vi "CheckLic.vi"() -> (0 "数据保存":bool, 1 "强制操作":bool, 2 "LicCode":string, 3 "机器码":string, 4 "参数生成":bool, 5 "参数配置":bool, 8 "鉴权通过":bool)   [LabVIEW 2013]
panel:
  out "子字符串":string
  out "Tip":string
  out "注册码":string
  out "连接的字符串":string
  in  "退出":bool
  in  "注册":bool
  in  "簇":T1
  out "字符串":string
  out "Times":dbl
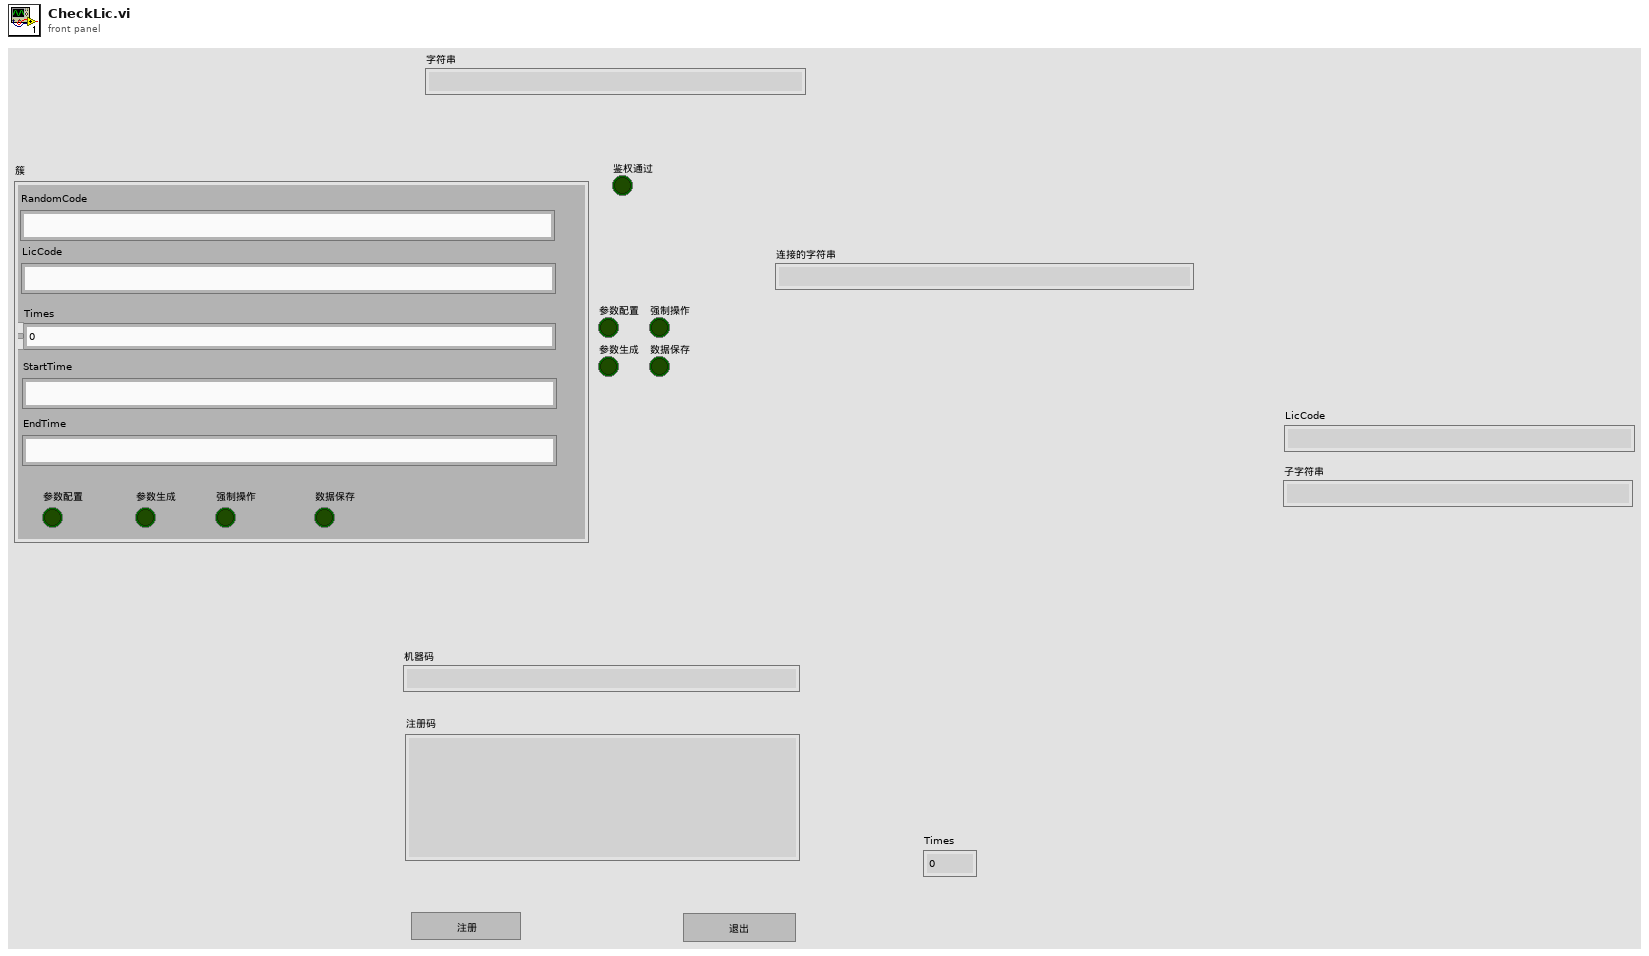
[diagram p1: front panel]
types:
  T1 = cluster{"RandomCode":string, "LicCode":string, "Times":dbl, "StartTime":string, "EndTime":string, "参数配置":bool, "参数生成":bool, "强制操作":bool, "数据保存":bool}
  T2 = enum32{"Invalid", "Standard", "Closed", "Hidden", "Minimized", "Maximized"}
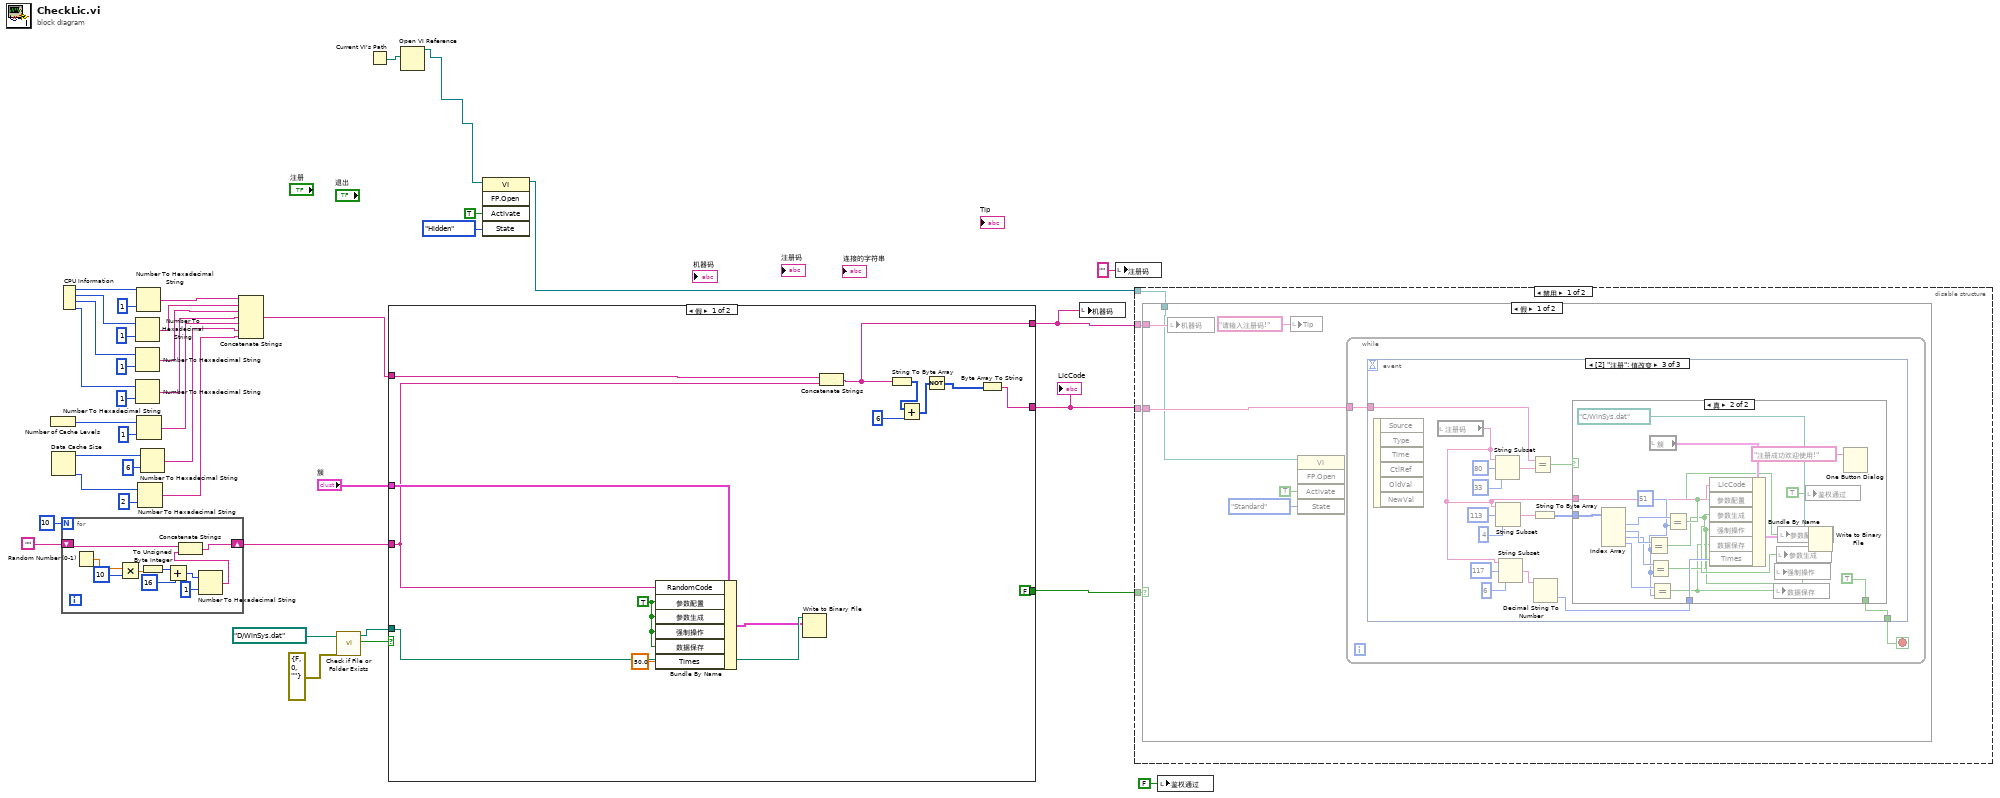
[diagram p0: block diagram]
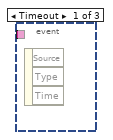
[diagram p2: hidden frame]
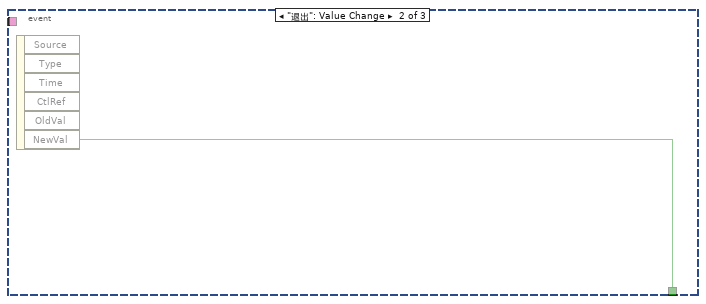
[diagram p3: hidden frame]
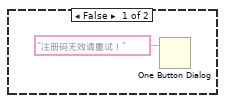
[diagram p4: hidden frame]
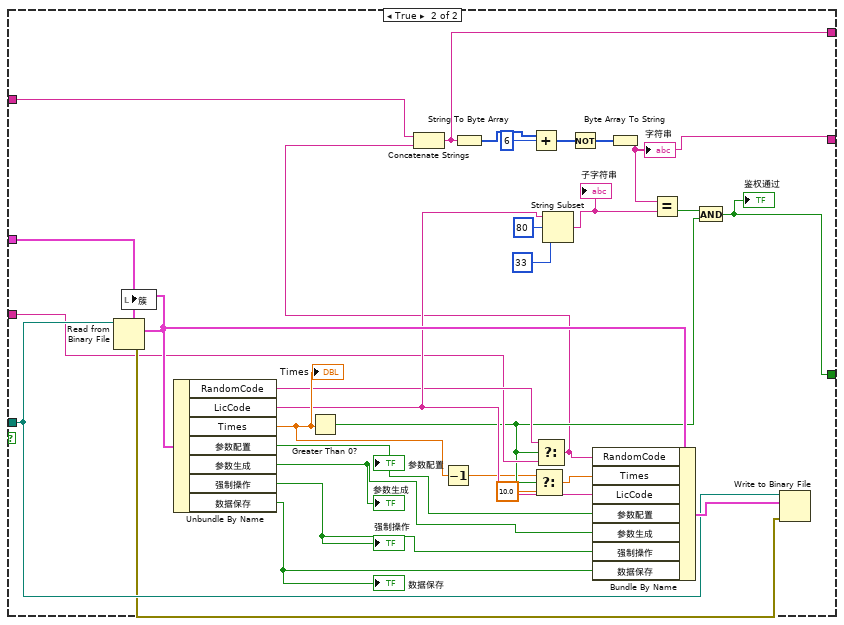
[diagram p7: hidden frame]
diagram:
  n1 = Number of Cache Levels() -> (w25:i32)
  n2 = Data Cache Size() -> (4:w26:i32, 7:w28:i32)  [unwired: 1 in]
  n3 = CPU Information() -> (4:w16:i32, 5:w20:i32, 6:w21:i32, 7:w22:i32)
  n4 = for {
    N: 10 -> [_]
    shift-right: [w42] -> w1
    shift-left: "" -> [w43]
    n5 = Random Number (0-1)() -> (number: 0 to 1=w50:dbl)
    n6 = Multiply(x=w50, y=u8 10) -> (x*y=w48:dbl)
    n7 = To Unsigned Byte Integer(number=w48) -> (unsigned 8bit integer=w46:u8)
    n8 = Add(x=w46, y=u8 16) -> (x+y=w44:u8)
    n9 = Number To Hexadecimal String(1:i16 1 ("宽度(-)"), 2:w44) -> (0:w41:string)
    n10 = Concatenate Strings(w43, w41) -> (w42:string)
  }
  n11 = Number To Hexadecimal String(1:i16 1 ("宽度(-)"), 2:w20) -> (0:w30:string)
  n12 = Number To Hexadecimal String(1:i16 1 ("宽度(-)"), 2:w21) -> (0:w31:string)
  n13 = Number To Hexadecimal String(1:i16 1 ("宽度(-)"), 2:w22) -> (0:w32:string)
  n14 = Number To Hexadecimal String(1:i16 1 ("宽度(-)"), 2:w16) -> (0:w29:string)
  n15 = Number To Hexadecimal String(1:i16 1 ("宽度(-)"), 2:w25) -> (0:w33:string)
  n16 = Number To Hexadecimal String(1:i16 2 ("宽度(-)"), 2:w28) -> (0:w35:string)
  n17 = Number To Hexadecimal String(1:i16 6 ("宽度(-)"), 2:w26) -> (0:w34:string)
  n18 = Concatenate Strings(w29, w30, w31, w32, w33, w34, w35) -> (w14:string)
  n19 = call <vilib>:"Check if File or Folder Exists.vi"("error in (no error)"=errorcluster {"status"=FALSE, "code"=0, "source"=""}, "path"=path "D:/WinSys.dat" ("文件（使用对话框）")) -> ("file or folder exists?"=w38:bool, "dup path"=w37:path)  [unwired: 7 in, 1 out]
  n20 = Current VI's Path() -> (path=w10:path)
  n21 = case shown="假" w38 {
    tunnel: w37 -> [w63 w79]
    tunnel: "簇" -> [w61 w92]
    tunnel: w14 -> [w58 w89]
    tunnel: [FALSE w83] -> w13
    tunnel: [w54 w82] -> w12
    tunnel: [w53 w81] -> w5
    tunnel: w1 -> [w52 w69]
    frame False {
      w60 = TRUE ("参数配置")
      n22 = Bundle By Name(cluster=w61, "RandomCode"=w52, "参数配置"=w60, "参数生成"=w60, "强制操作"=w60, "数据保存"=w60, "Times"=50.0) -> (w62:T1)
      n23 = Write to Binary File(file (use dialog)=w63, data=w62) -> ()  [unwired: 4 in, 3 out]
      n24 = Concatenate Strings(w58, w52) -> (w53:string)
      n25 = String To Byte Array(string=w53) -> (unsigned byte array=w57:u8[])
      n26 = Add(x=w57, y=u8 6) -> (x+y=w55:u8[])
      n27 = Not(x=w55) -> ()  [unwired: 1 out]
      n28 = Byte Array To String(unsigned byte array=w55) -> (string=w54:string)
    }
    frame True {
      n29 = Read from Binary File(5:w92, 11:w79) -> (0:w71:errorcluster, 2:w78:T1)  [unwired: 4 in, 2 out]
      n30 = local write "簇"(w78) -> ()
      n31 = Unbundle By Name(w78) -> ("RandomCode"=w70:string, "LicCode"=w72:string, "Times"=w77:dbl, "参数配置"=w76:bool, "参数生成"=w75:bool, "强制操作"=w74:bool, "数据保存"=w73:bool)
      "参数配置" <- w76
      "参数生成" <- w75
      "强制操作" <- w74
      "数据保存" <- w73
      "Times" <- w77
      n32 = Greater Than 0?(x=w77) -> (x > 0?=w68:bool)
      n33 = Decrement(x=w77) -> (x-1=w66:dbl)
      n34 = Select(t=w66, s=w68, f=10.0) -> (s? t:f=w67:dbl)
      n35 = Select(t=w70, s=w68, f=w69) -> (s? t:f=w64:string)
      n36 = Concatenate Strings(w89, w64) -> (w81:string)
      n37 = String To Byte Array(string=w81) -> (unsigned byte array=w88:u8[])
      n38 = Add(x=w88, y=u8 6) -> (x+y=w86:u8[])
      n39 = String Subset(string=w72, offset (0)=80 ("偏移量(0)"), length (rest)=33 ("长度（剩余）")) -> (substring=w85:string)
      "子字符串" <- w85
      n40 = Not(x=w86) -> ()  [unwired: 1 out]
      n41 = Bundle By Name(cluster=w78, "RandomCode"=w64, "Times"=w67, "LicCode"=w72, "参数配置"=w76, "参数生成"=w75, "强制操作"=w74, "数据保存"=w73) -> (w80:T1)
      n42 = Byte Array To String(unsigned byte array=w86) -> (string=w82:string)
      "字符串" <- w82
      n43 = Equal?(x=w82, y=w85) -> (x = y?=w84:bool)
      n44 = And(x=w84, y=w68) -> (x .and. y?=w83:bool)
      "鉴权通过" <- w83
      n45 = Write to Binary File(file (use dialog)=w79, data=w80, error in=w71) -> ()  [unwired: 3 in, 3 out]
    }
  }
  "LicCode" <- w12
  n46 = Open VI Reference(vi path=w10) -> (vi reference=w7:refnum<vi>)  [unwired: 5 in, 1 out]
  n47 = invoke class="VI" method="FP.Open"(reference=w7, "Activate"=TRUE ("激活？"), "State"=T2."Hidden" ("状态")) -> (reference out=w6:refnum<vi>)  [unwired: 2 in, 4 out]
  n48 = local write "机器码"(w5) -> ()
  n49 = local write "注册码"("" ("注册码")) -> ()
  n50 = disable-structure shown="禁用" {
    disable-tunnel: w13 -> [w96 _]
    disable-tunnel: w12 -> [w95 _]
    disable-tunnel: w5 -> [w94 _]
    disable-tunnel: w6 -> [w93 _]
    frame Disabled {
      n51 = case shown="假" w96 {
        tunnel: w95 -> [w102 _]
        tunnel: w94 -> [w100 _]
        tunnel: w93 -> [w97 _]
        frame False {
          n52 = local write "机器码"(w100) -> ()
          n53 = local write "Tip"("请输入注册码!" ("Tip")) -> ()
          n54 = invoke class="VI" method="FP.Open"(reference=w97, "Activate"=TRUE ("激活？"), "State"=T2."Standard" ("状态")) -> ()  [unwired: 2 in, 5 out]
          n55 = while {
            tunnel: w102 -> [w104]
            stop <- w103 stop-if-true
            n56 = event shown="[2] \"注册\": 值改变" {
              selector: _ -> [_ _ _]
              dyn-events: _ -> [_ _ _]
              timeout: _ -> [_ _ _]
              tunnel: w104 -> [_ _ w117]
              tunnel: [_ w105 w106] -> w103
              event Timeout {
                n57 = event-data() -> ()  [unwired: 1 in, 3 out]
              }
              event "退出": Value Change {
                n58 = event-data() -> ("NewVal"=w105:bool)  [unwired: 1 in, 5 out]
              }
              event "注册": Value Change {
                n59 = event-data() -> ()  [unwired: 1 in, 6 out]
                n60 = local read "注册码"() -> (w109:string)
                n61 = String Subset(string=w109, offset (0)=80 ("偏移量(0)"), length (rest)=33 ("长度（剩余）")) -> (substring=w120:string)
                n62 = String Subset(string=w109, offset (0)=113 ("偏移量(0)"), length (rest)=4 ("长度（剩余）")) -> (substring=w113:string)
                n63 = String Subset(string=w109, offset (0)=117 ("偏移量(0)"), length (rest)=6 ("长度（剩余）")) -> (substring=w108:string)
                n64 = Equal?(x=w117, y=w120) -> (x = y?=w116:bool)
                n65 = String To Byte Array(string=w113) -> (unsigned byte array=w112:u8[])
                n66 = Decimal String To Number(string=w108) -> (number=w107:i32)  [unwired: 2 in, 1 out]
                n67 = case shown="真" w116 {
                  tunnel: w112 -> [_ w136]
                  tunnel: w109 -> [_ w130]
                  tunnel: w107 -> [_ w129]
                  tunnel: [_ TRUE ("新值")] -> w106
                  frame False {
                    n68 = One Button Dialog(message="注册码无效请重试！" ("消息")) -> ()  [unwired: 1 in, 1 out]
                  }
                  frame True {
                    w131 = 51 ("索引")
                    n69 = Index Array(array=w136) -> (element #1=w135:u8, element #2=w134:u8, element #3=w133:u8, element #4=w132:u8)  [unwired: 4 in]
                    n70 = Equal?(x=w134, y=w131) -> (x = y?=w124:bool)
                    n71 = Equal?(x=w133, y=w131) -> (x = y?=w123:bool)
                    n72 = local read "簇"() -> (w137:T1)
                    n73 = Equal?(x=w132, y=w131) -> (x = y?=w122:bool)
                    n74 = Equal?(x=w135, y=w131) -> (x = y?=w125:bool)
                    n75 = Bundle By Name(cluster=w137, "LicCode"=w130, "参数配置"=w125, "参数生成"=w124, "强制操作"=w123, "数据保存"=w122, "Times"=w129) -> (w139:T1)
                    n76 = local write "数据保存"(w122) -> ()
                    n77 = local write "强制操作"(w123) -> ()
                    n78 = local write "参数生成"(w124) -> ()
                    n79 = local write "参数配置"(w125) -> ()
                    n80 = local write "鉴权通过"(TRUE ("鉴权通过")) -> ()
                    n81 = Write to Binary File(file (use dialog)=path "C:/WinSys.dat" ("文件（使用对话框）"), data=w139) -> ()  [unwired: 4 in, 3 out]
                    n82 = One Button Dialog(message="注册成功欢迎使用!" ("消息")) -> ()  [unwired: 1 in, 1 out]
                  }
                }
              }
            }
          }
        }
        frame True {
        }
      }
    }
    frame Enabled {
    }
  }
  n83 = local write "鉴权通过"(FALSE ("鉴权通过")) -> ()
